vi "CreateToolbarObject.vi"(0 "reference in":refnum<class "ClassDiagramGraph.lvclass">, 2 "GraphButton":u32, 5 "error in (no error)":errorcluster) -> (14 "reference out":refnum<class "ClassDiagramGraph.lvclass">, 15 "toolType":T1, 16 "Edge":refnum<class "AbstractEdge.lvclass">, 17 "Node":refnum<class "AbstractNode.lvclass">, 18 "ButtonNameCompressed)":string, 19 "error out":errorcluster)   [LabVIEW 2014, in "ClassDiagramGraph.lvclass"]
uses:
  <resource>/Framework/Providers/Open_GDS/UML/ClassDiagramGraph_class/ClassDiagramGraph.lvclass
  <resource>/Framework/Providers/Open_GDS/UML/UMLEditor/UMLEditor tooltype.ctl
  <resource>/Framework/Providers/Open_GDS/UML/AbstractEdge_class/AbstractEdge.lvclass
  <resource>/Framework/Providers/Open_GDS/UML/AbstractNode_class/AbstractNode.lvclass
  <resource>/Framework/Providers/Open_GDS/UML/ArrowHead_class/ArrowHeadType.ctl
  <resource>/Framework/Providers/Open_GDS/UML/BentStyle_class/BentStyleType.ctl
  <resource>/Framework/Providers/Open_GDS/UML/LineStyle_class/LineStyleType.ctl
  <resource>/Framework/Providers/Open_GDS/UML/Graph_class/ToolbarButtonType.ctl
  <resource>/Framework/Providers/Open_GDS/UML/Graphics_class/StrokeType.ctl
  <resource>/Framework/Providers/Open_GDS/UML/GeneralPathEdge_class/GeneralPathEdge.lvclass
  <resource>/Framework/Providers/Open_GDS/UML/RectangularNode_class/RectangularNode.lvclass
  <resource>/Framework/Providers/Open_GDS/UML/ClassRelationshipEdge_class/ClassRelationshipEdge.lvclass
  <resource>/Framework/Providers/Open_GDS/UML/Graph_class/Graph.lvclass
  <resource>/Framework/Providers/Open_GDS/UML/Graphics_class/Graphics.lvclass
  <resource>/Framework/Providers/Open_GDS/UML/ArrowHead_class/ArrowHead.lvclass
  <resource>/Framework/Providers/Open_GDS/UML/BentStyle_class/BentStyle.lvclass
  <resource>/Framework/Providers/Open_GDS/UML/SegmentedLineEdge_class/SegmentedLineEdge.lvclass
  <resource>/Framework/Providers/Open_GDS/UML/NoteEdge_class/NoteEdge.lvclass
  <resource>/Framework/Providers/Open_GDS/UML/LineStyle_class/LineStyle.lvclass
  <resource>/Framework/Providers/Open_GDS/UML/NoteNode_class/NoteNode.lvclass
  <resource>/Framework/Providers/Open_GDS/UML/PackageNode_class/PackageNode.lvclass
  <resource>/Framework/Providers/Open_GDS/UML/InterfaceNode_class/InterfaceNode.lvclass
  <resource>/Framework/Providers/Open_GDS/UML/ClassNode_class/ClassNode.lvclass
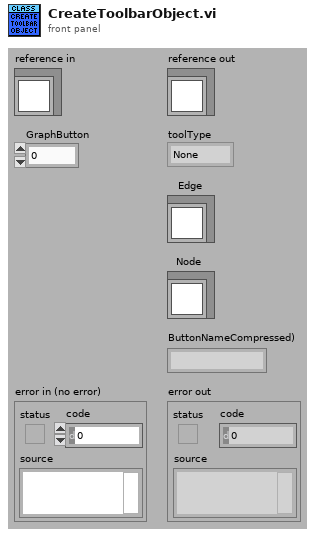
[diagram p1: front panel]
types:
  T1 = typedef "UMLEditor tooltype.ctl" = enum16{"None", "Node", "Edge"}
  T2 = typedef "LineStyle.lvclass/LineStyleType.ctl" = enum16{"SOLID", "DOTTED"}
  T3 = typedef "BentStyle.lvclass/BentStyleType.ctl" = enum16{"STRAIGHT", "HV", "VH", "HVH", "VHV", "ARC"}
  T4 = typedef "ArrowHead.lvclass/ArrowHeadType.ctl" = enum16{"NONE", "TRIANGLE", "BLACK_TRIANGLE", "V", "HALF_V", "DIAMOND", "BLACK_DIAMOND"}
  T5 = typedef "Graph.lvclass/ToolbarButtonType.ctl" = cluster{"Text":string, "Type":T1}
  T6 = typedef "Graphics.lvclass/StrokeType.ctl" = enum16{"USE_DEFAULT", "SOLID", "DOTTED"}
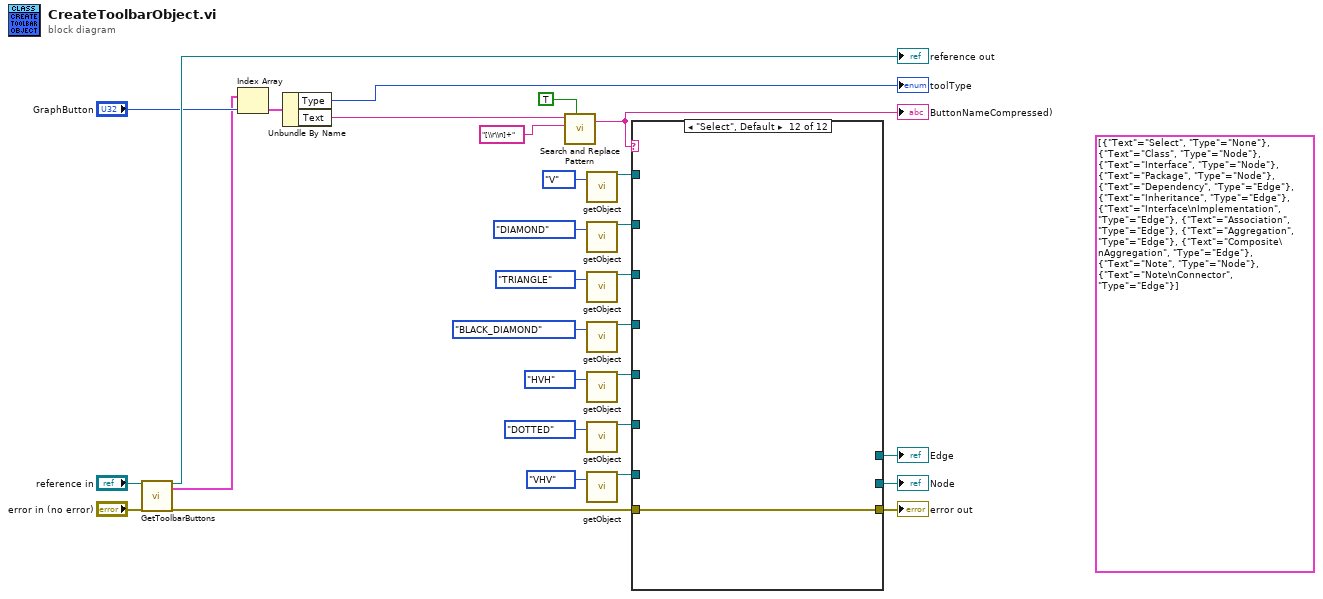
[diagram p0: block diagram]
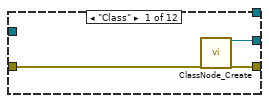
[diagram p2: hidden frame]
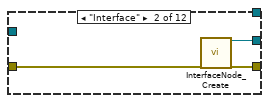
[diagram p3: hidden frame]
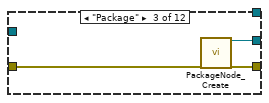
[diagram p4: hidden frame]
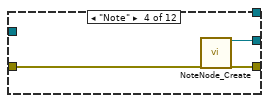
[diagram p5: hidden frame]
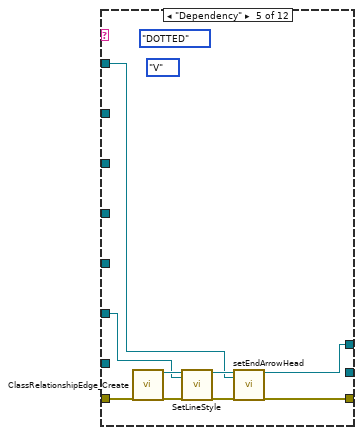
[diagram p6: hidden frame]
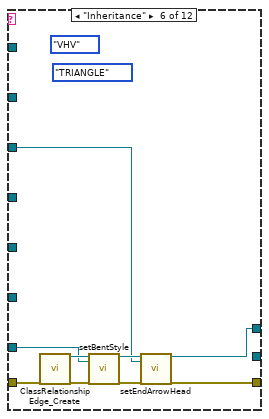
[diagram p7: hidden frame]
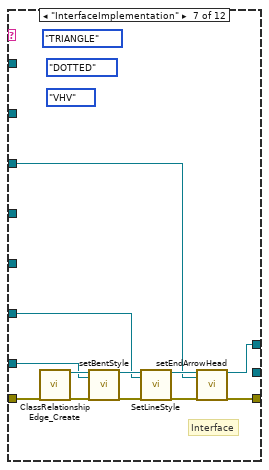
[diagram p8: hidden frame]
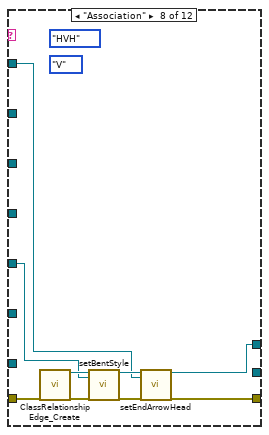
[diagram p9: hidden frame]
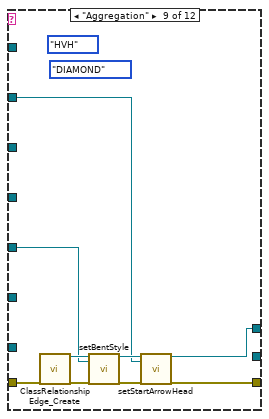
[diagram p10: hidden frame]
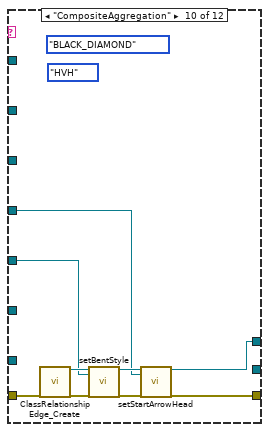
[diagram p11: hidden frame]
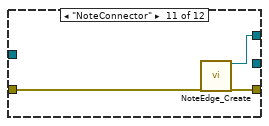
[diagram p12: hidden frame]
diagram:
  (unwired) T5[] [{"Text"="Select", "Type"=enum."None"}, {"Text"="Class", "Type"=enum."Node"}, {"Text"="Interface", "Type"=enum."Node"}, {"Text"="Package", "Type"=enum."Node"}, {"Text"="Dependency", "Type"=enum."Edge"}, {"Text"="Inheritance", "Type"=enum."Edge"}, {"Text"="Interface\nImplementation", "Type"=enum."Edge"}, {"Text"="Association", "Type"=enum."Edge"}, {"Text"="Aggregation", "Type"=enum."Edge"}, {"Text"="Composite\nAggregation", "Type"=enum."Edge"}, {"Text"="Note", "Type"=enum."Node"}, {"Text"="Note\nConnector", "Type"=enum."Edge"}] ("ToolbarButtons")
  n1 = call-dynamic "GetToolbarButtons.vi"("reference in"="reference in", "error in (no error)"="error in (no error)") -> ("reference out"=→"reference out":refnum<class "ClassDiagramGraph.lvclass">, "ToolbarButtons"=w20:T5[], "error out"=w12:errorcluster)  [unwired: 13 in, 2 out]
  n2 = Index Array(array=w20, index="GraphButton") -> (element=w1:T5)
  n3 = Unbundle By Name(w1) -> ("Type"=→"toolType":T1, "Text"=w4:string)
  n4 = call <vilib>:"Search and Replace Pattern.vi"("string"=w4, "regular expression (\"\")"="[\\r\\n]+" ("regular expression (\"\")"), "replace all? (F)"=TRUE) -> ("result string"=w21:string)  [unwired: 2 in, 1 out]
  "ButtonNameCompressed)" <- w21
  n5 = call <resource>:"getObject.vi"("arrowHead"=ArrowHeadType."V") -> ("reference out"=w10:refnum<class "ArrowHead.lvclass">)  [unwired: 1 in, 17 out]
  n6 = call <resource>:"getObject.vi"("arrowHead"=ArrowHeadType."DIAMOND") -> ("reference out"=w6:refnum<class "ArrowHead.lvclass">)  [unwired: 1 in, 17 out]
  n7 = call <resource>:"getObject.vi"("arrowHead"=ArrowHeadType."TRIANGLE") -> ("reference out"=w8:refnum<class "ArrowHead.lvclass">)  [unwired: 1 in, 17 out]
  n8 = call <resource>:"getObject.vi"("arrowHead"=ArrowHeadType."BLACK_DIAMOND") -> ("reference out"=w5:refnum<class "ArrowHead.lvclass">)  [unwired: 1 in, 17 out]
  n9 = call <resource>:"getObject.vi"("bentStyle"=BentStyleType."HVH") -> ("reference out"=w7:refnum<class "BentStyle.lvclass">)  [unwired: 1 in, 17 out]
  n10 = call <resource>:"getObject.vi"("lineStyle"=LineStyleType."DOTTED") -> ("reference out"=w11:refnum<class "LineStyle.lvclass">)  [unwired: 1 in, 17 out]
  n11 = call <resource>:"getObject.vi"("bentStyle"=BentStyleType."VHV") -> ("reference out"=w9:refnum<class "BentStyle.lvclass">)  [unwired: 1 in, 17 out]
  n12 = case shown="\"Select\", Default" w21 {
    tunnel: w12 -> [w32 w35 w36 w41 w48 w57 w65 w76 w85 w96 w101 w102]
    tunnel: [w31 w34 w38 w40 w45 w54 w64 w75 w84 w93 w100 w102] -> w28
    tunnel: [w30 w33 w37 w39 _ _ _ _ _ _ _ _] -> w23
    tunnel: w11 -> [_ _ _ _ w44 _ w62 _ _ _ _ _]
    tunnel: w10 -> [_ _ _ _ w43 _ _ w73 _ _ _ _]
    tunnel: w9 -> [_ _ _ _ _ w53 w63 _ _ _ _ _]
    tunnel: w8 -> [_ _ _ _ _ w52 w61 _ _ _ _ _]
    tunnel: w7 -> [_ _ _ _ _ _ _ w74 w83 w92 _ _]
    tunnel: w6 -> [_ _ _ _ _ _ _ _ w82 _ _ _]
    tunnel: w5 -> [_ _ _ _ _ _ _ _ _ w91 _ _]
    tunnel: [_ _ _ _ w42 w51 w60 w72 w81 w90 w99 _] -> w22
    frame "Class" {
      n13 = call <resource>:"ClassNode_Create.vi"("error in (no error)"=w32) -> ("reference out"=w30:refnum<class "ClassNode.lvclass">, "error out"=w31:errorcluster)  [unwired: 1 in, 16 out]
    }
    frame "Interface" {
      n14 = call <resource>:"InterfaceNode_Create.vi"("error in (no error)"=w35) -> ("reference out"=w33:refnum<class "InterfaceNode.lvclass">, "error out"=w34:errorcluster)  [unwired: 1 in, 16 out]
    }
    frame "Package" {
      n15 = call <resource>:"PackageNode_Create.vi"("error in (no error)"=w36) -> ("reference out"=w37:refnum<class "PackageNode.lvclass">, "error out"=w38:errorcluster)  [unwired: 1 in, 16 out]
    }
    frame "Note" {
      n16 = call <resource>:"NoteNode_Create.vi"("error in (no error)"=w41) -> ("reference out"=w39:refnum<class "NoteNode.lvclass">, "error out"=w40:errorcluster)  [unwired: 1 in, 16 out]
    }
    frame "Dependency" {
      (unwired) ArrowHeadType."V" ("arrowHead")
      (unwired) StrokeType."DOTTED" ("lineStyle")
      n17 = call <resource>:"ClassRelationshipEdge_Create.vi"("error in (no error)"=w48) -> ("reference out"=w49:refnum<class "ClassRelationshipEdge.lvclass">, "error out"=w47:errorcluster)  [unwired: 1 in, 16 out]
      n18 = call-dynamic "SetLineStyle.vi"("reference"=w49, "lineStyle"=w44, "error in (no error)"=w47) -> ("reference out"=w50:refnum<class "ClassRelationshipEdge.lvclass">, "error out"=w46:errorcluster)  [unwired: 15 in]
      n19 = call-dynamic "setEndArrowHead.vi"("reference"=w50, "endArrowHead"=w43, "error in (no error)"=w46) -> ("reference out"=w42:refnum<class "ClassRelationshipEdge.lvclass">, "error out"=w45:errorcluster)  [unwired: 15 in]
    }
    frame "Inheritance" {
      (unwired) BentStyleType."VHV" ("bentStyle")
      (unwired) ArrowHeadType."TRIANGLE" ("arrowHead")
      n20 = call <resource>:"ClassRelationshipEdge_Create.vi"("error in (no error)"=w57) -> ("reference out"=w59:refnum<class "ClassRelationshipEdge.lvclass">, "error out"=w56:errorcluster)  [unwired: 1 in, 16 out]
      n21 = call <resource>:"setBentStyle.vi"("reference"=w59, "newBentStyle"=w53, "error in (no error)"=w56) -> ("reference out"=w58:refnum<class "ClassRelationshipEdge.lvclass">, "error out"=w55:errorcluster)  [unwired: 15 out]
      n22 = call-dynamic "setEndArrowHead.vi"("reference"=w58, "endArrowHead"=w52, "error in (no error)"=w55) -> ("reference out"=w51:refnum<class "ClassRelationshipEdge.lvclass">, "error out"=w54:errorcluster)  [unwired: 15 in]
    }
    frame "InterfaceImplementation" {
      (unwired) StrokeType."DOTTED" ("lineStyle")
      (unwired) BentStyleType."VHV" ("bentStyle")
      (unwired) ArrowHeadType."TRIANGLE" ("arrowHead")
      # "Interface"
      n23 = call <resource>:"ClassRelationshipEdge_Create.vi"("error in (no error)"=w65) -> ("reference out"=w66:refnum<class "ClassRelationshipEdge.lvclass">, "error out"=w67:errorcluster)  [unwired: 1 in, 16 out]
      n24 = call <resource>:"setBentStyle.vi"("reference"=w66, "newBentStyle"=w63, "error in (no error)"=w67) -> ("reference out"=w68:refnum<class "ClassRelationshipEdge.lvclass">, "error out"=w69:errorcluster)  [unwired: 15 out]
      n25 = call-dynamic "SetLineStyle.vi"("reference"=w68, "lineStyle"=w62, "error in (no error)"=w69) -> ("reference out"=w70:refnum<class "ClassRelationshipEdge.lvclass">, "error out"=w71:errorcluster)  [unwired: 15 in]
      n26 = call-dynamic "setEndArrowHead.vi"("reference"=w70, "endArrowHead"=w61, "error in (no error)"=w71) -> ("reference out"=w60:refnum<class "ClassRelationshipEdge.lvclass">, "error out"=w64:errorcluster)  [unwired: 15 in]
    }
    frame "Association" {
      (unwired) BentStyleType."HVH" ("bentStyle")
      (unwired) ArrowHeadType."V" ("arrowHead")
      n27 = call <resource>:"ClassRelationshipEdge_Create.vi"("error in (no error)"=w76) -> ("reference out"=w77:refnum<class "ClassRelationshipEdge.lvclass">, "error out"=w78:errorcluster)  [unwired: 1 in, 16 out]
      n28 = call <resource>:"setBentStyle.vi"("reference"=w77, "newBentStyle"=w74, "error in (no error)"=w78) -> ("reference out"=w79:refnum<class "ClassRelationshipEdge.lvclass">, "error out"=w80:errorcluster)  [unwired: 15 out]
      n29 = call-dynamic "setEndArrowHead.vi"("reference"=w79, "endArrowHead"=w73, "error in (no error)"=w80) -> ("reference out"=w72:refnum<class "ClassRelationshipEdge.lvclass">, "error out"=w75:errorcluster)  [unwired: 15 in]
    }
    frame "Aggregation" {
      (unwired) ArrowHeadType."DIAMOND" ("arrowHead")
      (unwired) BentStyleType."HVH" ("bentStyle")
      n30 = call <resource>:"ClassRelationshipEdge_Create.vi"("error in (no error)"=w85) -> ("reference out"=w86:refnum<class "ClassRelationshipEdge.lvclass">, "error out"=w87:errorcluster)  [unwired: 1 in, 16 out]
      n31 = call <resource>:"setBentStyle.vi"("reference"=w86, "newBentStyle"=w83, "error in (no error)"=w87) -> ("reference out"=w88:refnum<class "ClassRelationshipEdge.lvclass">, "error out"=w89:errorcluster)  [unwired: 15 out]
      n32 = call <resource>:"setStartArrowHead.vi"("reference"=w88, "arroeHead"=w82, "error in (no error)"=w89) -> ("reference out"=w81:refnum<class "ClassRelationshipEdge.lvclass">, "error out"=w84:errorcluster)  [unwired: 15 out]
    }
    frame "CompositeAggregation" {
      (unwired) ArrowHeadType."BLACK_DIAMOND" ("arrowHead")
      (unwired) BentStyleType."HVH" ("bentStyle")
      n33 = call <resource>:"ClassRelationshipEdge_Create.vi"("error in (no error)"=w96) -> ("reference out"=w97:refnum<class "ClassRelationshipEdge.lvclass">, "error out"=w95:errorcluster)  [unwired: 1 in, 16 out]
      n34 = call <resource>:"setBentStyle.vi"("reference"=w97, "newBentStyle"=w92, "error in (no error)"=w95) -> ("reference out"=w98:refnum<class "ClassRelationshipEdge.lvclass">, "error out"=w94:errorcluster)  [unwired: 15 out]
      n35 = call <resource>:"setStartArrowHead.vi"("reference"=w98, "arroeHead"=w91, "error in (no error)"=w94) -> ("reference out"=w90:refnum<class "ClassRelationshipEdge.lvclass">, "error out"=w93:errorcluster)  [unwired: 15 out]
    }
    frame "NoteConnector" {
      n36 = call <resource>:"NoteEdge_Create.vi"("error in (no error)"=w101) -> ("reference out"=w99:refnum<class "NoteEdge.lvclass">, "error out"=w100:errorcluster)  [unwired: 1 in, 16 out]
    }
    frame "Select", Default {
    }
  }
  "error out" <- w28
  "Edge" <- w22
  "Node" <- w23
